vi "delay sincro.vi"(7 "milliseconds to wait":u32, 10 "error out":errorcluster, 11 "VISA resource name":refnum<visa-resource-name>) -> (2 "error out 2":errorcluster, 3 "VISA resource name 2":refnum<visa-resource-name>)   [LabVIEW 2019]
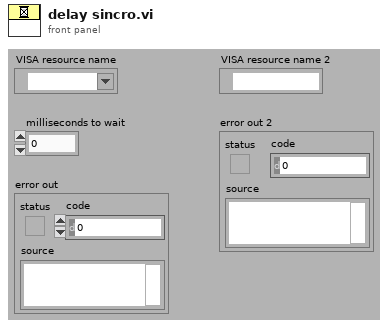
[diagram p1: front panel]
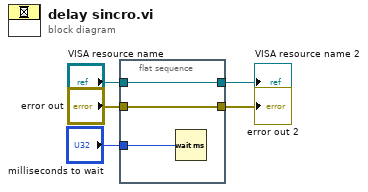
[diagram p0: block diagram]
diagram:
  n1 = flat-sequence {
    tunnel: [w8] -> w1
    tunnel: "VISA resource name" -> [w8]
    tunnel: [w7] -> w3
    tunnel: "error out" -> [w7]
    tunnel: "milliseconds to wait" -> [w6]
    frame #0 {
      n2 = Wait (ms)(milliseconds to wait=w6) -> ()  [unwired: 1 out]
    }
  }
  "error out 2" <- w3
  "VISA resource name 2" <- w1
